vi "Disconnect.vi"(8 "error in (no error)":errorcluster, 11 "4300 in":refnum<class "4300.lvclass">) -> (0 "error out":errorcluster, 3 "4300 out":refnum<class "4300.lvclass">)   [LabVIEW 2019, in "4300.lvlib" / "4300.lvclass"]
uses:
  Library/4300.lvclass
  Library/4300.lvclass/4300.ctl
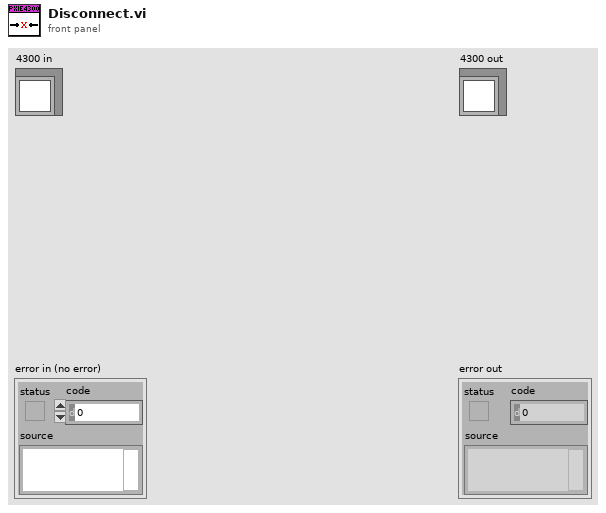
[diagram p1: front panel]
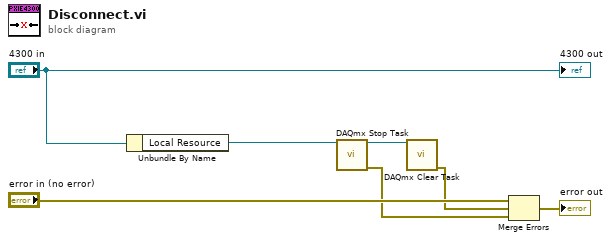
[diagram p0: block diagram]
diagram:
  n1 = Unbundle By Name("4300 in") -> ("Local Resource"=w5:refnum<k21>)
  n2 = call <vilib>:"DAQmx Stop Task.vi"("task/channels in"=w5) -> ("task out"=w4:refnum<k21>, "error out"=w3:errorcluster)  [unwired: 13 in]
  n3 = call <vilib>:"DAQmx Clear Task.vi"("task in"=w4) -> ("error out"=w1:errorcluster)  [unwired: 14 in]
  n4 = Merge Errors("error in (no error)", w1, w3) -> (→"error out":errorcluster)
  "4300 out" <- "4300 in"
